vi "pthread_cond_init.vi"(8 "error in (no error)":errorcluster, 10 "cond attr ptr in":u64, 11 "cond ptr in":u64) -> (0 "error out":errorcluster, 2 "cond attr ptr out":u64, 3 "cond ptr out":u64)   [LabVIEW 2013, in "Linux RT IPC.lvlib" / "POSIX Threads.lvlib" / "POSIX Thread Object.lvclass"]
uses:
  POSIX Thread Object.lvclass
  Controls/pthread functions.ctl
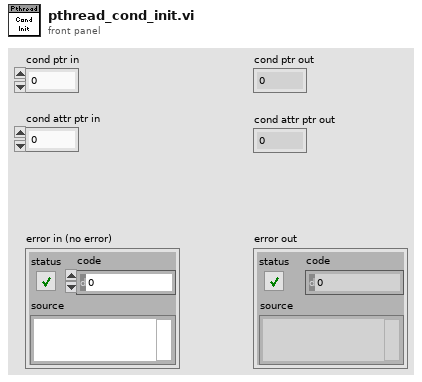
[diagram p1: front panel]
types:
  T1 = typedef "Linux RT IPC.lvlib/POSIX Threads.lvlib/POSIX Thread Object.lvclass/pthread functions.ctl" = enum16{"unspecified", "pthread_condattr_init", "pthread_condattr_destroy", "pthread_condattr_getclock", "pthread_condattr_setclock", "pthread_condattr_getpshared", "pthread_condattr_setpshared", "pthread_cond_init", "pthread_cond_destroy", "pthread_cond_broadcast", "pthread_cond_signal", "pthread_cond_timedwait", "pthread_cond_wait", "pthread_mutexattr_init", "pthread_mutexattr_destroy", "pthread_mutexattr_getprioceiling", "pthread_mutexattr_setprioceiling", "pthread_mutexattr_getprotocol", "pthread_mutexattr_setprotocol", "pthread_mutexattr_getpshared", "pthread_mutexattr_setpshared", "pthread_mutexattr_gettype", "pthread_mutexattr_settype", "pthread_mutex_init", "pthread_mutex_destroy", "pthread_mutex_getprioceiling", "pthread_mutex_setprioceiling", "pthread_mutex_lock", "pthread_mutex_timedlock", "pthread_mutex_trylock", "pthread_mutex_unlock", "sem_destroy", "sem_getvalue", "sem_init", "sem_post", "sem_timedwait", "sem_trywait", "sem_wait", "barrier_init", "barrier_destroy", "barrier_wait", "barrierattr_init", "barrierattr_destroy", "barrierattr_getpshared", "barrierattr_setpshared"}
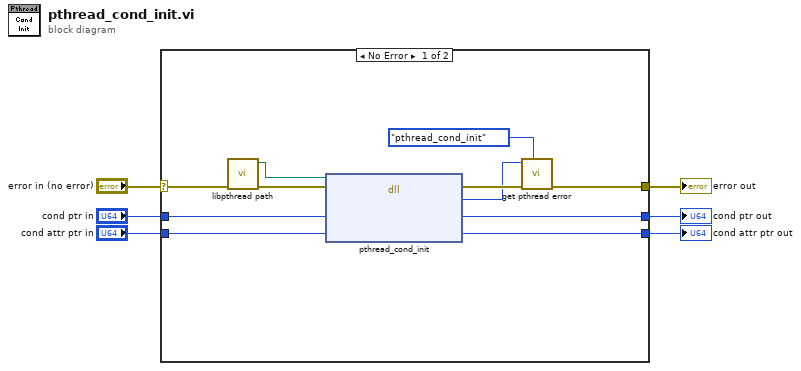
[diagram p0: block diagram]
diagram:
  n1 = case shown="No Error" "error in (no error)" {
    selector: "error in (no error)" -> [w17 w20]
    tunnel: "cond ptr in" -> [w16 w19]
    tunnel: [w15 w20] -> w4
    tunnel: "cond attr ptr in" -> [w14 w18]
    tunnel: [w13 w19] -> w2
    tunnel: [w12 w18] -> w1
    frame No Error {
      n2 = call "libpthread path.vi"("error in (no error)"=w17) -> ("error out"=w10:errorcluster, "path to libpthread"=w11:path)  [unwired: 9 in]
      n3 = dll-call lib="?" fn="pthread_cond_init"(path in=w11, error in=w10, "cond"=w16, "cond attr"=w14) -> (error out=w9:errorcluster, "errno"=w8:i32, "cond"=w13:u64, "cond attr"=w12:u64)  [unwired: 1 in, 1 out]
      n4 = call "get pthread error.vi"("function"=pthread_functions."pthread_cond_init", "error in (no error)"=w9, "errno"=w8) -> ("error out"=w15:errorcluster)  [unwired: 8 in]
    }
    frame Error {
    }
  }
  "error out" <- w4
  "cond ptr out" <- w2
  "cond attr ptr out" <- w1
